vi "Global1.vi"() -> ()   [LabVIEW 2019]
panel:
  out "Width":dbl=4.0
  out "Score":dbl
  in  "Get marks":dbl[](array[numeric])
  out "Speed":dbl
  in  "z":dbl[](array[numeric])
  in  "y":dbl[](array[numeric])
  in  "x":dbl[](array[numeric])
  out "Up \nUp":i32
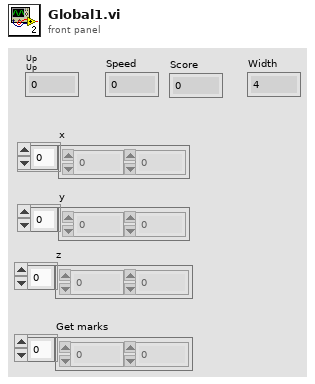
[diagram p1: front panel]
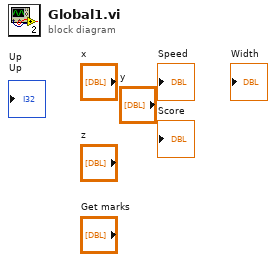
[diagram p0: block diagram]
diagram:
